vi "Interpolation Query.vi"(8 "error in":errorcluster, 11 "Instrument Handle In":i32) -> (0 "error out":errorcluster, 2 "Format":i32(ring) items=["None", "First", "Sinc"], 3 "Instrument Handle Out":i32)   [LabVIEW 8.6, in "ZTScopeM.lvlib"]
doc: "Query the waveform interpolation format."
uses:
  ZTScopeM.lvlib
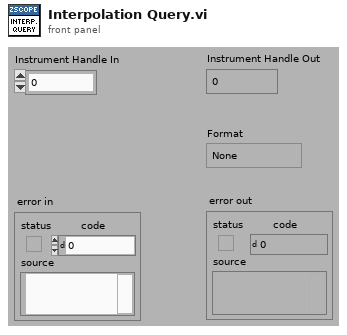
[diagram p1: front panel]
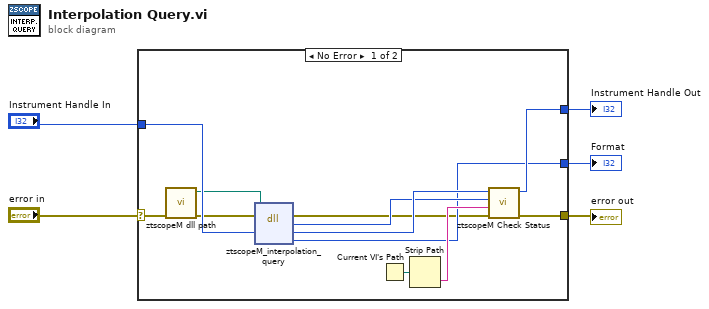
[diagram p0: block diagram]
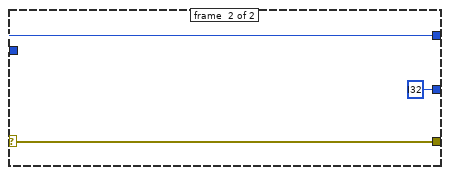
[diagram p2: hidden frame]
diagram:
  n1 = case shown="No Error" "error in" {
    selector: "error in" -> [w9 w20]
    tunnel: [w12 w20] -> w2
    tunnel: "Instrument Handle In" -> [w17 w19]
    tunnel: [w11 w19] -> w4
    tunnel: [w10 i32 ? ("format")] -> w1
    frame #0 {
      n2 = call "ztscopeM dll path.vi"("error in (no error)"=w9) -> ("error out"=w7:errorcluster, "<instrument>.dll path"=w8:path)  [unwired: 9 in]
      n3 = dll-call lib="C:/Program Files (x86)/National Instruments/LabVIEW 2013/instr.lib/ztscopem/ztscopeM.dll" fn="ztscopeM_interpolation_query"(path in=w8, error in=w7, "instrumentHandle"=w17) -> (error out=w6:errorcluster, w13:i32, "instrumentHandle"=w14:i32, "format"=w10:i32)  [unwired: 1 in, 2 out]
      n4 = Current VI's Path() -> (path=w16:path)
      n5 = Strip Path(path=w16) -> (name=w15:string)  [unwired: 1 out]
      n6 = call "ztscopeM Check Status.vi"("error in"=w6, "name of VI"=w15, "status (return code)"=w13, "instrument handle in"=w14) -> ("error out"=w12:errorcluster, "instrument handle out"=w11:i32)  [unwired: 2 out]
    }
    frame #1 {
    }
  }
  "Instrument Handle Out" <- w4
  "error out" <- w2
  "Format" <- w1
